vi "Web Control Multi-Example.vi"() -> ()   [LabVIEW 2026]
uses:
  <extravilib>/ChannelInstances/Tag-bool/Write With Abort.vi
  <extravilib>/ChannelInstances/Tag-bool/Read With Abort.vi
  <extravilib>/ChannelInstances/Tag-bool/Instantiate.vi
  <extravilib>/ChannelInstances/Tag-bool/EndpointRead.vi
  <extravilib>/ChannelInstances/Tag-bool/Endpoint.vi
  <vilib>/measure/NI_MABase.lvlib
  <extravilib>/ChannelInstances/Tag-bool.lvlib
panel:
  in  "Tree":string(tree)
  in  "Stop":bool
  out "Web Browser Control":string(html)="https://github.com/zeshanabdullah10/controlstack-web-bridge"
  out "Tab Control":T1(tab)
  in  "URL":string="https://maps.google.com"
  in  "Current Pole Zero Ratio":dbl(slide)=1.1445696004512624 scale=0.125..8.0
  in  "Current Compensation Freq":dbl(slide)=22308.395489073177 scale=300.0..250000.0 scale format="%#_6p"
  in  "Current Gain Bandwidth":dbl(slide)=284803.5868435805 scale=1000.0..1000000.0 scale format="%#_6p"
  out "Waveform Graph":waveform(dbl)[](graph)
  in  "Voltage Gain Bandwidth":dbl(slide)=31651.12089336408 scale=1000.0..50000.0 scale format="%#_6p"
  in  "Voltage Compensation Freq":dbl(slide)=6761.680050362442 scale=300.0..250000.0 scale format="%#_6p"
  in  "Voltage Pole Zero Ratio":dbl(slide)=1.1040895136738123 scale=0.125..8.0
  in  "GWeb Page":string="http://localhost:9090/nxgproxy/62653/HtmlVI/Build/VireoDevSystem/Interactive/WebApp.gcomp/index.html"
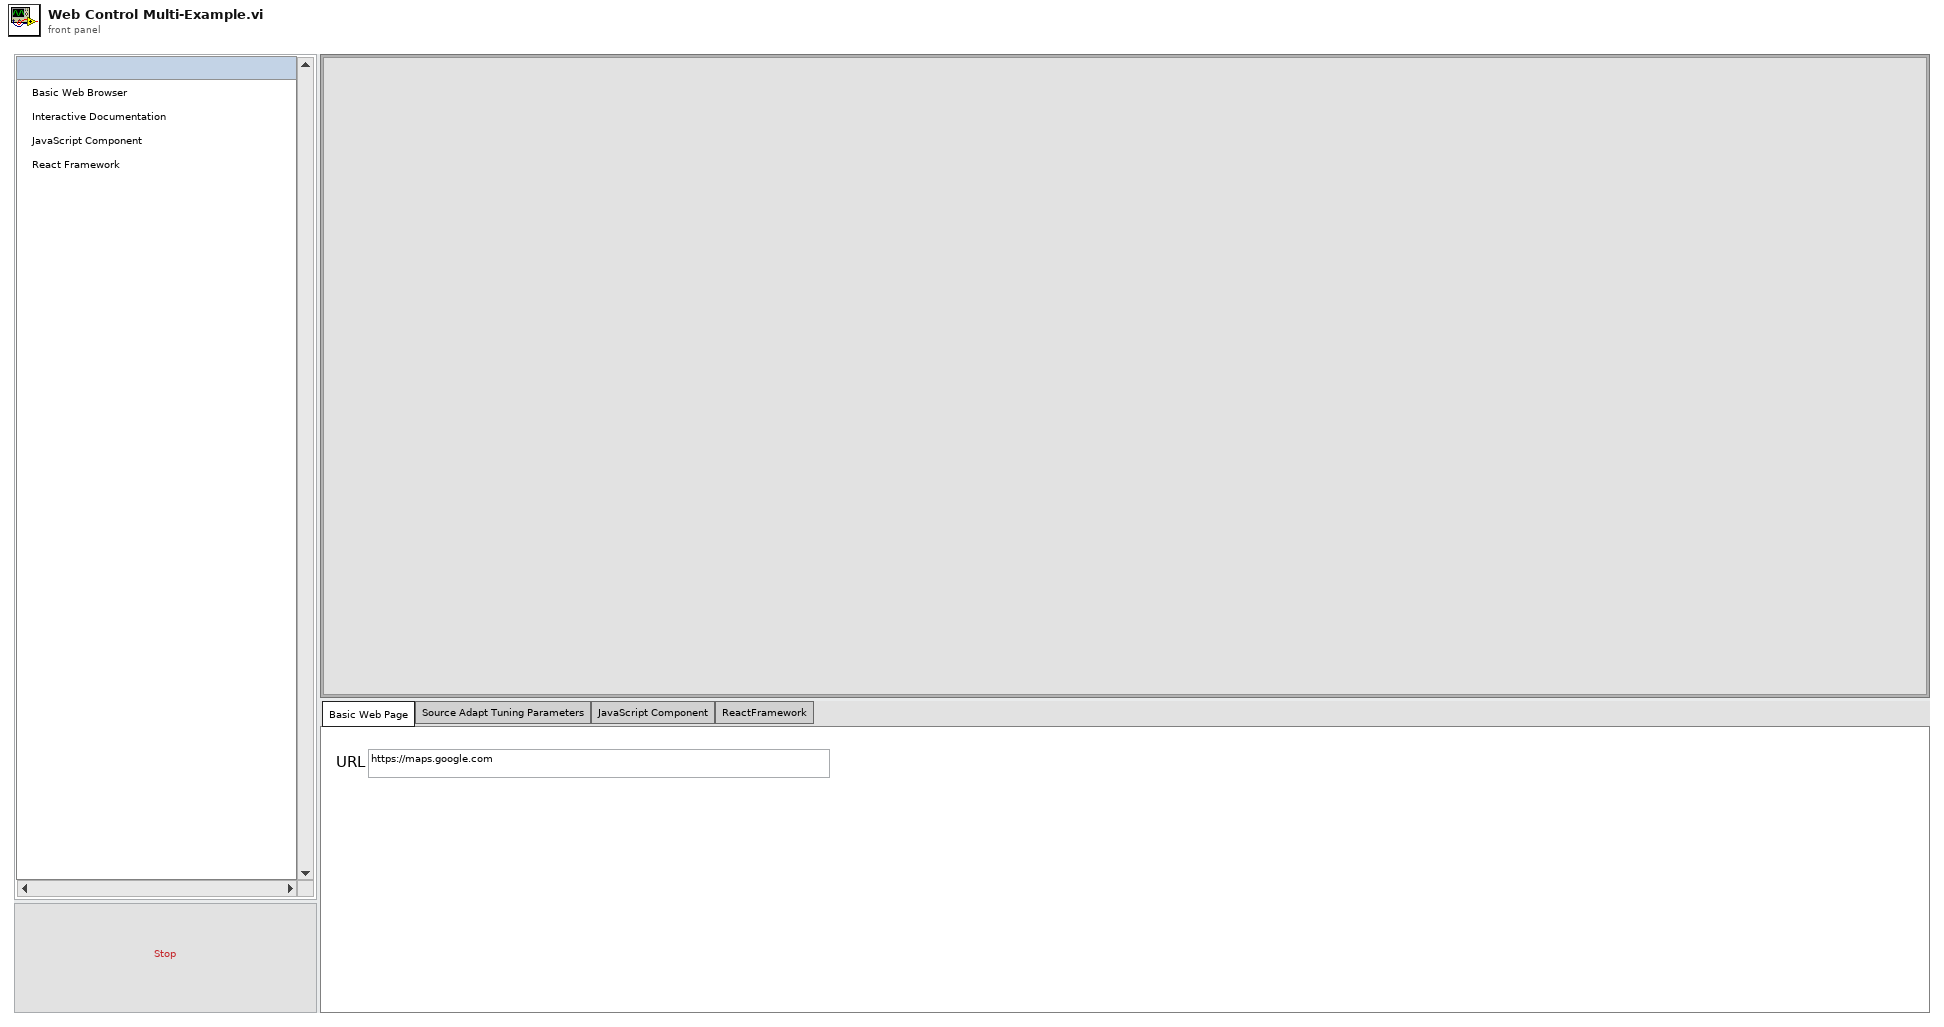
[diagram p1: front panel]
types:
  T1 = enum32{"Basic Web Page", "Source Adapt Tuning Parameters", "JavaScript Component", "ReactFramework"}
  T2 = typedef "Tag-bool.lvlib/))Channel.ctl" = refnum<queue>
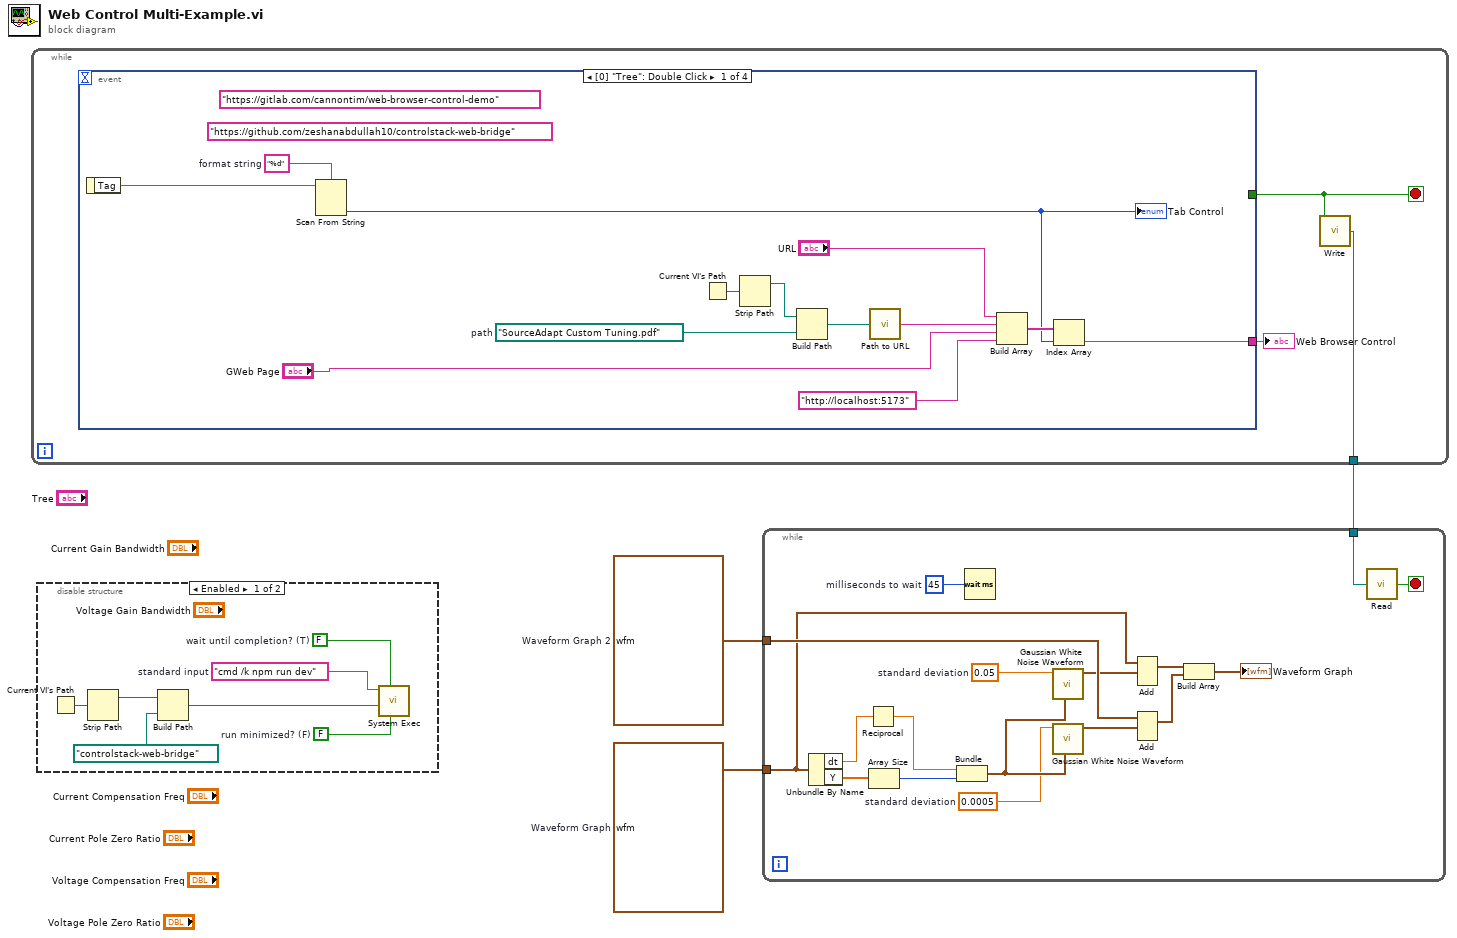
[diagram p0: block diagram]
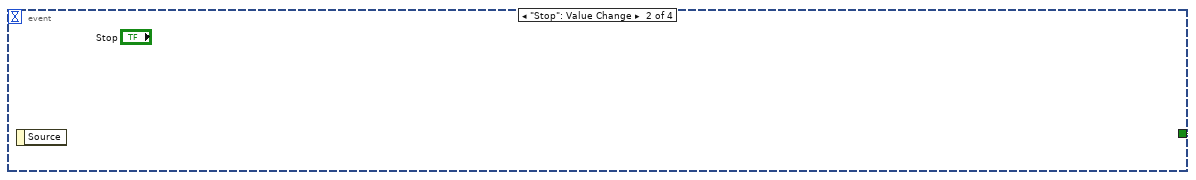
[diagram p2: hidden frame]
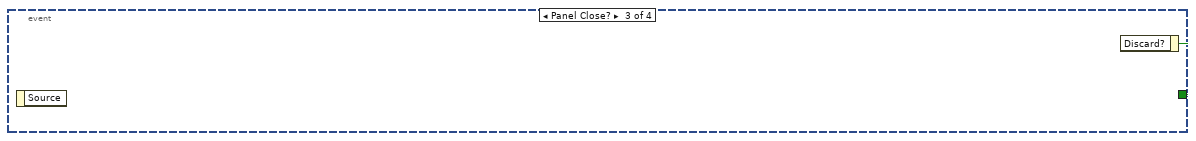
[diagram p3: hidden frame]
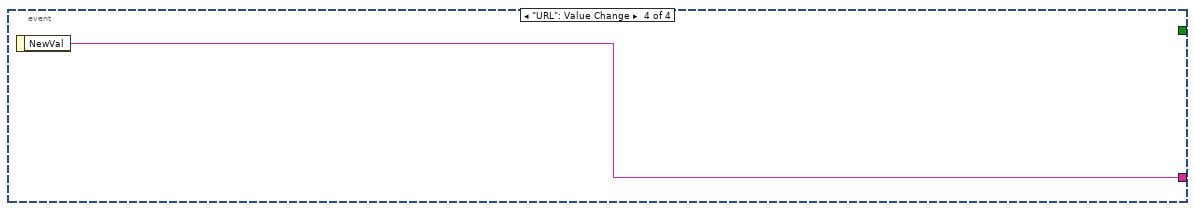
[diagram p4: hidden frame]
diagram:
  w2 = waveform(dbl) {"t0"=timestamp(0 s since 1904-01-01), "dt"=3.3333333333333333e-06, "Y"=array[500 elements]}  # Waveform Graph
  w3 = waveform(dbl) {"t0"=timestamp(0 s since 1904-01-01), "dt"=3.3333333333333333e-06, "Y"=array[500 elements]}  # Waveform Graph 2
  n1 = while {
    tunnel: [w4] -> w1
    stop <- w5 stop-if-true
    n2 = event shown="[0] \"Tree\": Double Click" {
      selector: _ -> [_ _ _ _]
      dyn-events: _ -> [_ _ _ _]
      timeout: _ -> [_ _ _ _]
      tunnel: [_ TRUE w21 _] -> w5
      tunnel: [w8 _ _ w22] -> w6
      event "Tree": Double Click {
        w11 = "%d"  # format string
        w18 = path "SourceAdapt Custom Tuning.pdf"  # path
        (unwired) "https://gitlab.com/cannontim/web-browser-control-demo"
        (unwired) "https://github.com/zeshanabdullah10/controlstack-web-bridge"
        n3 = event-data() -> ("Tag"=w12:string)  [unwired: 1 in]
        n4 = Scan From String(format string=w11, input string=w12) -> (output 1=w9:T1)  [unwired: 3 in, 3 out]
        "Tab Control" <- w9
        n5 = Current VI's Path() -> (path=w19:path)
        n6 = Strip Path(path=w19) -> (stripped path=w17:path)  [unwired: 1 out]
        n7 = Build Path(base path=w17, name or relative path=w18) -> (appended path=w16:path)
        n8 = call <vilib>:"Path to URL.vi"("path"=w16) -> ("url"=w14:string)
        n9 = Build Array("URL", w14, "GWeb Page", "http://localhost:5173") -> (w10:string[])
        n10 = Index Array(array=w10, index=w9) -> (element=w8:string)
      }
      event "Stop": Value Change {
        n11 = event-data() -> ()  [unwired: 1 in, 1 out]
      }
      event Panel Close? {
        w21 = TRUE
        n12 = event-data() -> ()  [unwired: 1 in, 1 out]
        n13 = event-data("Discard?"=w21) -> ()  [unwired: 1 in, 1 out]
      }
      event "URL": Value Change {
        n14 = event-data() -> ("NewVal"=w22:string)  [unwired: 1 in]
      }
    }
    "Web Browser Control" <- w6
    n15 = call <extravilib>:"Write.vi"("element"=w5) -> ("channel"=w4:T2)  [unwired: 1 out]
  }
  n16 = disable-structure shown="Enabled" {
    frame Enabled {
      w23 = "cmd /k npm run dev"  # standard input
      w28 = FALSE  # wait until completion? (T)
      w29 = FALSE  # run minimized? (F)
      n17 = Current VI's Path() -> (path=w27:path)
      n18 = Strip Path(path=w27) -> (stripped path=w26:path)  [unwired: 1 out]
      n19 = Build Path(base path=w26, name or relative path=path "controlstack-web-bridge") -> (appended path=w24:path)
      n20 = call <vilib>:"System Exec.vi"("run minimized? (F)"=w29, "wait until completion? (T)"=w28, "working directory"=w24, "command line"=w23) -> ()  [unwired: 4 in, 4 out]
    }
    frame Disabled {
    }
  }
  n21 = while {
    tunnel: w3 -> [w46]
    tunnel: w2 -> [w38]
    tunnel: w1 -> [w33]
    stop <- w32 stop-if-true
    w30 = u32 45  # milliseconds to wait
    w31 = 0.0005  # standard deviation
    w35 = 0.05  # standard deviation
    n22 = Unbundle By Name(w38) -> ("dt"=w43:dbl, "Y"=w41:dbl[])
    n23 = Reciprocal(x=w43) -> (1/x=w42:dbl)
    n24 = Array Size(array=w41) -> (size(s)=w40:i32)
    n25 = Bundle(w42, w40) -> (w36:cluster{dbl, i32})  [unwired: 1 in]
    n26 = Wait (ms)(milliseconds to wait=w30) -> ()  [unwired: 1 out]
    n27 = call <vilib>:"Gaussian White Noise Waveform.vi"("sampling info"=w36, "standard deviation"=w35) -> ("signal out"=w39:waveform(dbl))  [unwired: 8 in, 1 out]
    n28 = call <vilib>:"Gaussian White Noise Waveform.vi"("sampling info"=w36, "standard deviation"=w31) -> ("signal out"=w34:waveform(dbl))  [unwired: 8 in, 1 out]
    n29 = Add(1:w39, 2:w38) -> (0:w37:waveform(dbl))  [unwired: 1 in, 1 out]
    n30 = Add(1:w34, 2:w46) -> (0:w44:waveform(dbl))  [unwired: 1 in, 1 out]
    n31 = Build Array(w37, w44) -> (→"Waveform Graph":waveform(dbl)[])
    n32 = call <extravilib>:"Read.vi"("channel"=w33) -> ("element"=w32:bool)  [unwired: 1 in, 1 out]
  }
